vi "ADC (B).vi"(8 "error in":errorcluster, 11 "Adc":refnum<k24>) -> (0 "error out":errorcluster, 3 "Sample":dbl)   [LabVIEW 2011]
doc: "Control the analog/digital converter with constant values (basic version)"
uses:
  C:/Program Files/Metrohm Autolab/Autolab SDK 1.10/EcoChemie.Autolab.Sdk.dll
  EcoChemie.Autolab.Sdk.dll
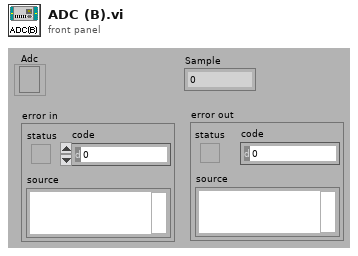
[diagram p1: front panel]
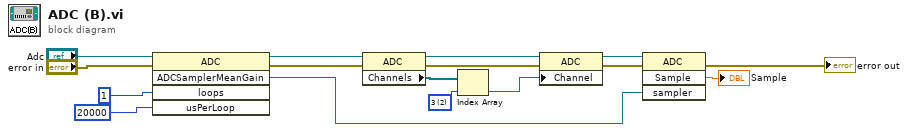
[diagram p0: block diagram]
diagram:
  w8 = 2 items=["16"=15, "15"=14, "14"=13, "13"=12, "12"=11, "11"=10, "10"=9, "9"=8, "8"=7, "7"=6, "6"=5, "5"=4, "4"=3, "3"=2, "2"=1, "1"=0] ("Channel")
  n1 = invoke class="ADC" method="ADCSamplerMeanGain"(reference="Adc", error in="error in", "loops"=1 ("Loops"), "usPerLoop"=u16 20000) -> (reference out=w3:refnum<k24>, error out=w4:errorcluster, "ADCSamplerMeanGain"=w5:refnum<k24>)  [unwired: 1 in, 2 out]
  n2 = property class="ADC"(reference=w3, error in=w4) -> (reference out=w16:refnum<k24>, error out=w15:errorcluster, "Channels"=w14:refnum<k24>[])
  n3 = Index Array(array=w14, index=w8) -> (element=w13:refnum<k24>)
  n4 = property class="ADC"(reference=w16, error in=w15, "Channel"=w13) -> (reference out=w12:refnum<k24>, error out=w11:errorcluster)
  n5 = invoke class="ADC" method="Sample"(reference=w12, error in=w11, "sampler"=w5) -> (error out=→"error out":errorcluster, "Sample"=→"Sample":dbl)  [unwired: 1 in, 2 out]
